vi "GetFileVersionInfo.vi"(8 "error in":errorcluster, 10 "Size":i32, 11 "lptstrFilename":string) -> (0 "error out":errorcluster, 3 "lpData":string)   [LabVIEW 2015]
doc: "The GetFileVersionInfo function retrieves version information for the specified file."
uses:
  version.dll
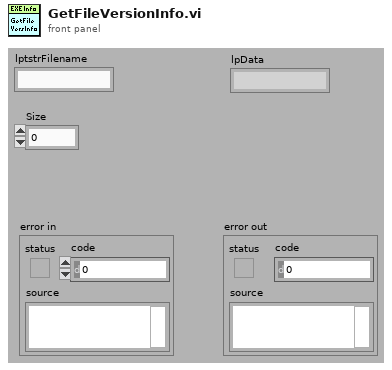
[diagram p1: front panel]
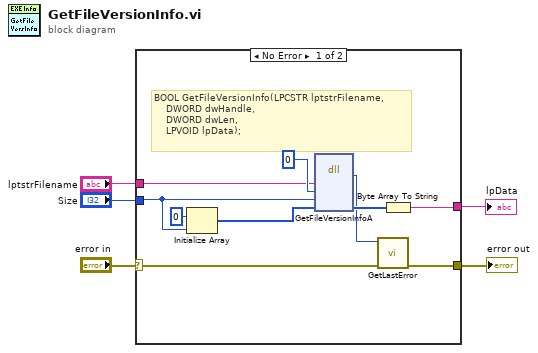
[diagram p0: block diagram]
diagram:
  n1 = case shown="No Error" "error in" {
    selector: "error in" -> [w9 w16]
    tunnel: [w6 _] -> w1
    tunnel: "lptstrFilename" -> [w12 _]
    tunnel: [w8 w16] -> w4
    tunnel: "Size" -> [w11 _]
    frame No Error {
      # "BOOL GetFileVersionInfo(LPCSTR lptstrFilename,\n    DWORD dwHandle,\n    DWORD dwLen,\n    LPVOID lpData);"
      n2 = Initialize Array(u8 0, w11) -> (w7:u8[])
      n3 = dll-call lib="version.dll" fn="GetFileVersionInfoA"("lptstrFilename"=w12, "dwhandle"=0, "dwlen"=w11, "lpData"=w7) -> (w10:i32, "lpData"=w13:u8[])  [unwired: 6 in, 2 out]
      n4 = call "GetLastError.vi"("error in (no error)"=w9, "Status"=w10) -> ("error out"=w8:errorcluster)  [unwired: 9 in]
      n5 = Byte Array To String(unsigned byte array=w13) -> (string=w6:string)
    }
    frame Error {
    }
  }
  "error out" <- w4
  "lpData" <- w1
